vi "Sequence.vi"() -> ()   [LabVIEW 2015]
panel:
  out "output array":string[](array[string])
  in  "stop":bool
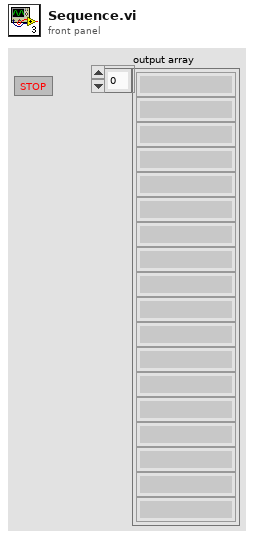
[diagram p1: front panel]
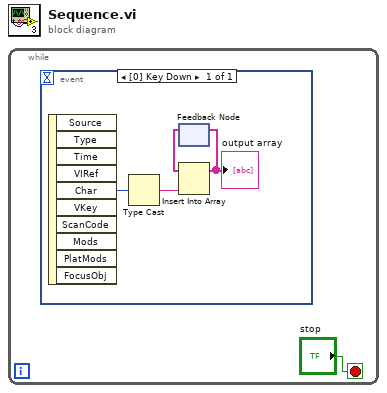
[diagram p0: block diagram]
diagram:
  n1 = while {
    stop <- "stop" stop-if-true
    n2 = event shown="[0] Key Down" {
      selector: _ -> [_]
      dyn-events: _ -> [_]
      timeout: _ -> [_]
      event Key Down {
        n3 = event-data() -> ("Char"=w3:i16)  [unwired: 1 in, 9 out]
        n4 = Type Cast(x=w3) -> (*(type *) &x=w2:string)  [unwired: 1 in]
        n5 = feedback #1() -> (w5:string[])  [unwired: 1 in]
        n6 = Insert Into Array(array=w5, new element=w2) -> (w4:string[])  [unwired: 1 in]
        "output array" <- w4
        n7 = feedback-in #1(w4) -> ()
      }
    }
  }
